vi "count laser stim photons.vi"(7 "count window":bool, 9 "read output":T1, 10 "stim on?":bool) -> (1 "n photons during stim":u32, 2 "stim time":u32)   [LabVIEW 2010]
uses:
  common_typedefs/channels_cluster.ctl
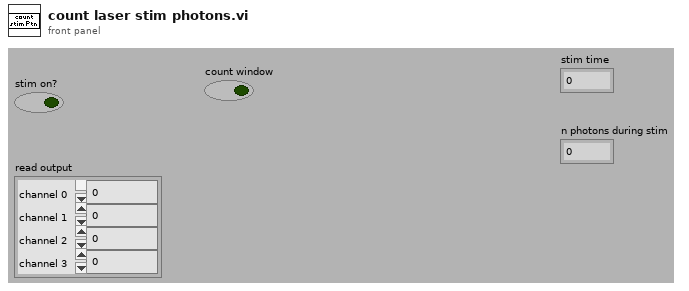
[diagram p1: front panel]
types:
  T1 = typedef "channels_cluster.ctl" = cluster{"channel 0":u32, "channel 1":u32, "channel 2":u32, "channel 3":u32}
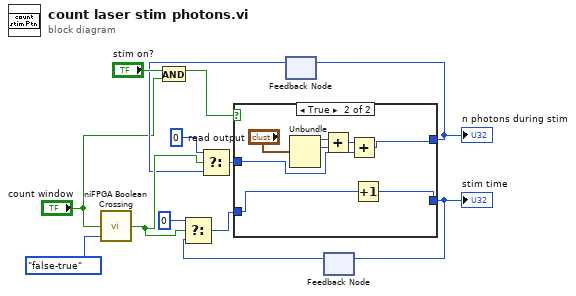
[diagram p0: block diagram]
diagram:
  n1 = call <vilib>:"niFPGA Boolean Crossing.vi"("input"="count window", "direction"=enum8{"either", "false-true", "true-false"}."false-true") -> ("crossing"=w6:bool)  [unwired: 7 in]
  n2 = And(x="stim on?", y="count window") -> (x .and. y?=w2:bool)
  n3 = feedback #1() -> (w3:u32)  [unwired: 1 in]
  n4 = Select(t=u32 0, s=w6, f=w3) -> (s? t:f=w4:u32)
  n5 = feedback #2() -> (w8:u32)  [unwired: 1 in]
  n6 = Select(t=u32 0, s=w6, f=w8) -> (s? t:f=w9:u32)
  n7 = case shown="True" w2 {
    tunnel: [w15 w19] -> w13
    tunnel: [w14 w18] -> w12
    tunnel: w9 -> [w14 w17]
    tunnel: w4 -> [w15 w16]
    frame False {
    }
    frame True {
      n8 = Unbundle("read output") -> ("channel 0"=w22:u32, "channel 1"=w21:u32)  [unwired: 2 out]
      n9 = Add(x=w22, y=w21) -> (x+y=w20:u32)
      n10 = Add(x=w20, y=w16) -> (x+y=w19:u32)
      n11 = Increment(x=w17) -> (x+1=w18:u32)
    }
  }
  "stim time" <- w12
  "n photons during stim" <- w13
  n12 = feedback-in #1(w13) -> ()
  n13 = feedback-in #2(w12) -> ()
